vi "ESP8266 UDP Server Writing Samples To Listeners.vi"() -> ()   [LabVIEW 2014]
uses:
  <vilib>/LabVIEW Universal Transcriptor/LabVIEW to Arduino Transcriptor/Transcriptors/System API/Serial println string.vi
  <vilib>/LabVIEW Universal Transcriptor/ESP8266 WiFi Wrapper/ESP8266 WiFi Wrapper.lvlib
  <vilib>/LabVIEW Universal Transcriptor/Arduino MPU6050 Library/Arduino MPU6050.lvlib
panel:
  out "Error Out":errorcluster
  in  "DNS address":u8[](array[numeric])=[0, 0, 0, 0]
  in  "IP address":u8[](array[numeric])=[192, 168, 0, 47]
  in  "Gateway":u8[](array[numeric])=[192, 168, 0, 1]
  in  "Subnet mask":u8[](array[numeric])=[255, 255, 255, 0]
  in  "Password":string="12345678"
  in  "SSID":string="ESP8266 Wifi UDP"
  in  "Listen Port":i16=8080
  in  "error in (no error)":errorcluster
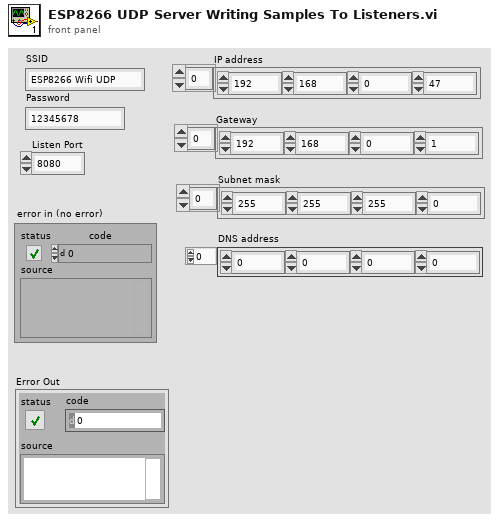
[diagram p1: front panel]
types:
  T1 = enum16{"MPU6050_SCALE_250DPS", "MPU6050_SCALE_500DPS", "MPU6050_SCALE_1000DPS", "MPU6050_SCALE_2000DPS"}
  T2 = enum16{"MPU6050_RANGE_2G", "MPU6050_RANGE_4G", "MPU6050_RANGE_8G", "MPU6050_RANGE_16G"}
  T3 = enum16{"WIFI_OFF", "WIFI_STA", "WIFI_AP", "WIFI_AP_STA"}
  T4 = typedef "Arduino MPU6050.lvlib/MPU6050LibVector.ctl" = cluster{"XAxis":sgl, "YAxis":sgl, "ZAxis":sgl}
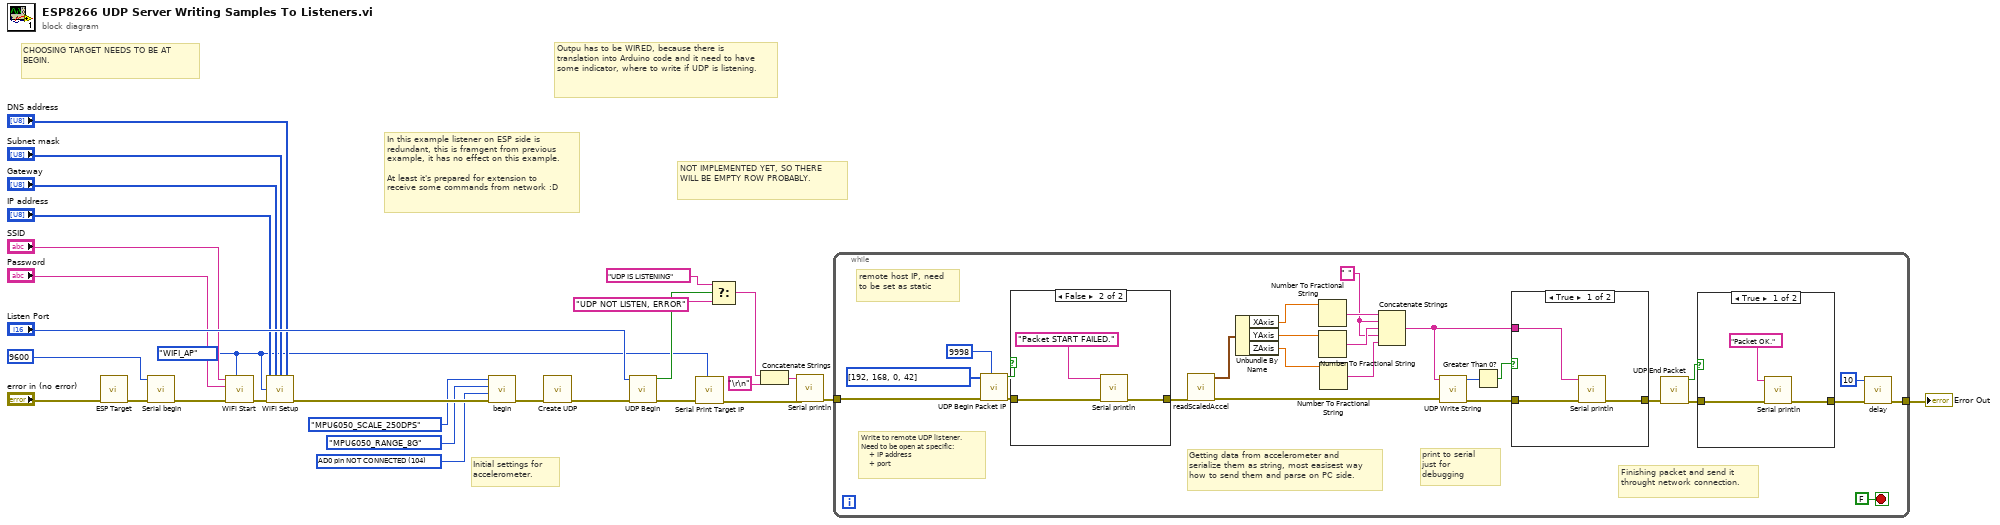
[diagram p0: block diagram]
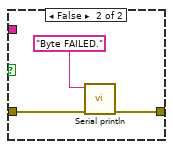
[diagram p2: hidden frame]
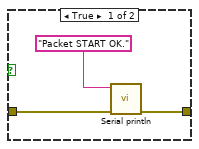
[diagram p3: hidden frame]
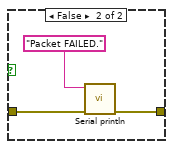
[diagram p4: hidden frame]
diagram:
  w3 = u16 104 items=["AD0 pin NOT CONNECTED"=104, "AD0 connect to Vcc"=105] ("address")
  w6 = T3."WIFI_AP" ("WiFi Mode")
  # "In this example listener on ESP side is redundant, this is framgent from previous example, it has no effect on this example.\n\nAt least it's prepared for extension to receive some commands from network :D"
  # "Initial settings for accelerometer."
  # "NOT IMPLEMENTED YET, SO THERE WILL BE EMPTY ROW PROBABLY."
  # "Outpu has to be WIRED, because there is translation into Arduino code and it need to have some indicator, where to write if UDP is listening."
  # "CHOOSING TARGET NEEDS TO BE AT BEGIN."
  n1 = call <vilib>:"ESP Target.vi"("Error In"="error in (no error)") -> ("Error Out"=w28:errorcluster)  [unwired: 10 in]
  n2 = call <vilib>:"Serial begin.vi"("Error In"=w28, "speed (Bd)"=u32 9600 ("Speed")) -> ("Error Out"=w19:errorcluster)  [unwired: 9 in]
  n3 = call <vilib>:"WiFi Start.vi"("WiFi Mode"=w6, "Error In"=w19, "Password"="Password", "SSID"="SSID") -> ("Error Out"=w18:errorcluster)  [unwired: 7 in]
  n4 = call <vilib>:"WiFi Setup.vi"("IP address"="IP address", "Gateway address"="Gateway", "Subnet mask"="Subnet mask", "DNS address"="DNS address", "WiFi Mode"=w6, "Error In"=w18) -> ("Error Out"=w5:errorcluster)  [unwired: 9 in]
  n5 = call <vilib>:"begin.vi"("Error In"=w5, "address"=w3, "range"=T2."MPU6050_RANGE_8G", "scale"=T1."MPU6050_SCALE_250DPS") -> ("Error Out"=w4:errorcluster)  [unwired: 7 in]
  n6 = call <vilib>:"Create UDP.vi"("Error In"=w4) -> ("Error Out"=w17:errorcluster)  [unwired: 10 in]
  n7 = call <vilib>:"UDP Begin.vi"("Error In"=w17, "Port"="Listen Port") -> ("Error Out"=w8:errorcluster, "Is listening?"=w13:bool)  [unwired: 8 in]
  n8 = call <vilib>:"Serial Print Target IP.vi"("WiFi Mode"=w6, "Error In"=w8) -> ("Error Out"=w7:errorcluster)  [unwired: 9 in]
  n9 = Select(t="UDP IS LISTENING", s=w13, f="UDP NOT LISTEN, ERROR") -> (s? t:f=w10:string)
  n10 = Concatenate Strings(w10, "\r\n") -> (w12:string)
  n11 = call-poly <vilib>:"Serial println.vi"("Error In"=w7, "string in"=w12) -> ("Error Out"=w16:errorcluster)  [unwired: 9 in]
  n12 = while {
    tunnel: w16 -> [w52]
    tunnel: [w53] -> w9
    stop <- FALSE stop-if-true
    w31 = " " ("string")
    # "print to serial just for debugging"
    # "remote host IP, need to be set as static"
    # "Finishing packet and send it throught network connection."
    # "Getting data from accelerometer and serialize them as string, most easisest way how to send them and parse on PC side."
    # "Write to remote UDP listener.\nNeed to be open at specific:\n    + IP address\n    + port"
    n13 = call <vilib>:"UDP Begin Packet IP.vi"("Port"=i16 9998, "Error In"=w52, "IP Address"=u8[] [192, 168, 0, 42]) -> ("Error Out"=w46:errorcluster, "Successful?"=w45:bool)  [unwired: 7 in]
    n14 = case shown="False" w45 {
      tunnel: w46 -> [w64 w67]
      tunnel: [w63 w66] -> w43
      frame True {
        n15 = call-poly <vilib>:"Serial println.vi"("Error In"=w64, "string in"="Packet START OK.") -> ("Error Out"=w63:errorcluster)  [unwired: 9 in]
      }
      frame False {
        n16 = call-poly <vilib>:"Serial println.vi"("Error In"=w67, "string in"="Packet START FAILED.") -> ("Error Out"=w66:errorcluster)  [unwired: 9 in]
      }
    }
    n17 = call <vilib>:"readScaledAccel.vi"("error in (no error)"=w43) -> ("error out"=w35:errorcluster, "Vector"=w42:T4)  [unwired: 9 in]
    n18 = Unbundle By Name(w42) -> ("XAxis"=w38:sgl, "YAxis"=w37:sgl, "ZAxis"=w36:sgl)
    n19 = Number To Fractional String(number=w38) -> (F-format string=w41:string)  [unwired: 3 in]
    n20 = Number To Fractional String(number=w37) -> (F-format string=w40:string)  [unwired: 3 in]
    n21 = Number To Fractional String(number=w36) -> (F-format string=w39:string)  [unwired: 3 in]
    n22 = Concatenate Strings(w41, w31, w40, w31, w39) -> (w30:string)
    n23 = call <vilib>:"UDP Write String.vi"("Error In"=w35, "String to write"=w30) -> ("Error Out"=w32:errorcluster, "Chars written"=w34:u8)  [unwired: 8 in]
    n24 = Greater Than 0?(x=w34) -> (x > 0?=w33:bool)
    n25 = case shown="True" w33 {
      tunnel: [w58 w61] -> w44
      tunnel: w32 -> [w56 w59]
      tunnel: w30 -> [w57 _]
      frame True {
        n26 = call-poly <vilib>:"Serial println.vi"("Error In"=w56, "string in"=w57) -> ("Error Out"=w58:errorcluster)  [unwired: 9 in]
      }
      frame False {
        n27 = call-poly <vilib>:"Serial println.vi"("Error In"=w59, "string in"="Byte FAILED.") -> ("Error Out"=w61:errorcluster)  [unwired: 9 in]
      }
    }
    n28 = call <vilib>:"UDP End Packet.vi"("Error In"=w44) -> ("Error Out"=w50:errorcluster, "Successful?"=w48:bool)  [unwired: 9 in]
    n29 = case shown="True" w48 {
      tunnel: w50 -> [w70 w73]
      tunnel: [w69 w72] -> w49
      frame True {
        n30 = call-poly <vilib>:"Serial println.vi"("Error In"=w70, "string in"="Packet OK.") -> ("Error Out"=w69:errorcluster)  [unwired: 9 in]
      }
      frame False {
        n31 = call-poly <vilib>:"Serial println.vi"("Error In"=w73, "string in"="Packet FAILED.") -> ("Error Out"=w72:errorcluster)  [unwired: 9 in]
      }
    }
    n32 = call <vilib>:"delay.vi"("Error In"=w49, "time (ms)"=10) -> ("Error Out"=w53:errorcluster)  [unwired: 9 in]
  }
  "Error Out" <- w9
